vi "NM GlobalTest.vi"() -> ()   [LabVIEW 2010] (continued)
  in  "data 21":digitalwaveform[](array[waveform])
  in  "sDWrite":T7(tab)
  in  "data 22":bool
  in  "data 23":bool[](array[boolean])
  in  "data 24":u8 format="%x"
  in  "data 25":u16 format="%x"
  in  "data 26":u32 format="%x"
  in  "data 27":digitalwaveform(waveform)={"t0"=timestamp(0 s since 1904-01-01), "dt"=0.0, "Y"={"transitions"=[], "data"=[]}, "error"={"status"=FALSE, "code"=37421928, "source"=""}}
  out "data 28":u8[](array[numeric])
  out "data 29":u16[](array[numeric]) format="%x"
  out "data 30":u32[](array[numeric]) format="%x"
  in  "data 31":digitalwaveform(waveform)={"t0"=timestamp(0 s since 1904-01-01), "dt"=0.0, "Y"={"transitions"=[], "data"=[]}, "error"={"status"=FALSE, "code"=37421928, "source"=""}}
  in  "nOrsCChan":enum32{"Multi-Channel", "Single Channel"}(tab)=enum."Single Channel"
  in  "nCtrWrite":enum32{"Frequency", "Time", "Ticks"}(tab)
  in  "data 32":cluster{"duty cycle":dbl, "frequency":dbl}[](array[cluster])
  in  "data 34":cluster{"high time":dbl, "low time":dbl}[](array[cluster])
  in  "data 33":cluster{"high ticks":u32, "low ticks":u32}[](array[cluster])
  in  "sCtrWrite":enum32{"Frequency", "Time", "Ticks"}(tab)
  in  "frequency":dbl=1.0 format="%_6g"
  in  "duty cycle":dbl=0.5 format="%_6g"
  in  "high time":dbl=0.01 format="%_6g"
  in  "low time":dbl=0.01 format="%_6g"
  in  "high ticks":u32=100
  in  "low ticks":u32=100
  in  "CompWrite":enum32{"2D", "1D Waveform"}(tab)
  out "DblArray 2":dbl[][](array[numeric])
  out "u32Array":u32[][](array[numeric])
  out "DblPlot":dbl[][](graph)
  out "u32Plot":u32[][](graph)
  in  "Plots":bool
  in  "digital data 2":digitalwaveform[](array[waveform])
  out "WfmArray":waveform(dbl)[](array[waveform])
  in  "Write":bool
  in  "SelLib":enum32{"ULx", "DAQmx"}(tab)
  out "NumberOfChannels":u32
  out "Task":i32 format="%x"
  out "ToString":string
  out "ChanType":i32(ring)=10100 items=["Analog Input"=10100, "Analog Output"=10102, "Digital Input"=10151, "Digital Output"=10153, "Counter Input"=10131, "Counter Output"=10132]
  out "Name":refnum<k21>
  in  "Task Control Action":i32(ring)=2 items=["verify"=2, "reserve"=4, "commit"=3, "unreserve"=5, "abort"=6]
  in  "TaskType":T10(tab)
  in  "AChan":enum32{"ULx", "DAQmx"}(tab)
  in  "AnalogType":T11(tab)
  in  "min 3":dbl=-5.0
  in  "max 3":dbl=5.0
  in  "min 2":dbl=-5.0
  in  "max 2":dbl=5.0
  in  "min":dbl=-5.0
  in  "max":dbl=5.0
  in  "physical channels 3":refnum<k21>
  in  "physical channels 2":refnum<k21>
  in  "ULx":refnum<k21>
  in  "min 5":dbl=-0.01 format="%_4f"
  in  "max 5":dbl=0.01 format="%_4g"
  in  "min 4":dbl=-0.01 format="%_4f"
  in  "max 4":dbl=0.01 format="%_4g"
  in  "min":dbl=-0.01 format="%_4f"
  in  "max":dbl=0.01 format="%_4g"
  in  "physical channels 6":refnum<k21>
  in  "physical channels 5":refnum<k21>
  in  "ULx":refnum<k21>
  in  "units 3":i32(ring) items=["degC", "degF", "kelvin", "raw"]
  in  "units 2":i32(ring) items=["degC", "degF", "kelvin", "raw"]
  in  "units":i32(ring) items=["degC", "degF", "kelvin", "raw"]
  in  "physical channels 9":refnum<k21>
  in  "physical channels 8":refnum<k21>
  in  "ULx":refnum<k21>
  in  "physical channels 12":refnum<k21>
  in  "min 7":dbl=-5.0
  in  "max 7":dbl=5.0
  in  "physical channels 11":refnum<k21>
  in  "min 8":dbl=-5.0
  in  "max 8":dbl=5.0
  in  "min":dbl=-5.0
  in  "max":dbl=5.0
  in  "ULx":refnum<k21>
  in  "min 10":dbl=-10.0
  in  "max 10":dbl=10.0
  in  "min 11":dbl=-10.0
  in  "max 11":dbl=10.0
  in  "min":dbl=-10.0
  in  "max":dbl=10.0
  in  "physical channels 15":refnum<k21>
  in  "physical channels 14":refnum<k21>
  in  "ULx":refnum<k21>
  in  "xAnalog\nType":T11(tab)
  in  "physical channels 33":tag
  in  "physical channels 32":tag
  in  "DAQmx":tag
  in  "min 20":dbl=-5.0
  in  "max 20":dbl=5.0
  in  "min 19":dbl=-5.0
  in  "max 19":dbl=5.0
  in  "min":dbl=-5.0
  in  "max":dbl=5.0
  in  "name 1":string
  in  "name 2":string
  in  "name 3":string
  in  "physical channels 36":tag
  in  "physical channels 35":tag
  in  "min 23":dbl=-0.01 format="%0.5f"
  in  "max 23":dbl=0.01 format="%0.5f"
  in  "min 22":dbl=-0.01 format="%0.5f"
  in  "max 22":dbl=0.01 format="%0.5f"
  in  "min":dbl=-0.01 format="%0.5f"
  in  "max":dbl=0.01 format="%0.5f"
  in  "DAQmx":tag
  in  "units 15":i32(ring)=10143 items=["Deg C"=10143, "Deg F"=10144, "Kelvins"=10325, "Deg R"=10145, "From Custom Scale"=10065]
  in  "units 13":i32(ring)=10143 items=["Deg C"=10143, "Deg F"=10144, "Kelvins"=10325, "Deg R"=10145, "From Custom Scale"=10065]
  in  "min 26":dbl format="%0.2f"
  in  "max 26":dbl=100.0 format="%0.2f"
  in  "min 25":dbl format="%0.2f"
  in  "max 25":dbl=100.0 format="%0.2f"
  in  "min":dbl format="%0.2f"
  in  "max":dbl=100.0 format="%0.2f"
  in  "physical channels 39":tag
  in  "physical channels 38":tag
  in  "units":i32(ring)=10143 items=["Deg C"=10143, "Deg F"=10144, "Kelvins"=10325, "Deg R"=10145, "From Custom Scale"=10065]
  in  "DAQmx":tag
  in  "Names":string
  in  "T2":string
  in  "T3":string
  in  "min 29":dbl=-10.0 format="%0.2f"
  in  "max 29":dbl=10.0 format="%0.2f"
  in  "min 28":dbl=-10.0 format="%0.2f"
  in  "max 28":dbl=10.0 format="%0.2f"
  in  "min":dbl=-10.0 format="%0.2f"
  in  "max":dbl=10.0 format="%0.2f"
  in  "physical channels 42":tag
  in  "physical channels 41":tag
  in  "DAQmx":tag
  in  "physical channels 45":tag
  in  "physical channels 44":tag
  in  "min 32":dbl format="%0.5f"
  in  "max 32":dbl=0.02 format="%0.5f"
  in  "min 31":dbl format="%0.5f"
  in  "max 31":dbl=0.02 format="%0.5f"
  in  "min":dbl format="%0.5f"
  in  "max":dbl=0.02 format="%0.5f"
  in  "DAQmx":tag
  in  "DChan":enum32{"ULx", "DAQmx"}(tab)
  in  "DigitalType":enum32{"Digital Input", "Digital Output"}(tab)
  in  "line grouping 3":i32(ring)=1 items=["OneChannelForEachLine", "OneChannelForAllLines"]
  in  "line grouping 2":i32(ring)=1 items=["OneChannelForEachLine", "OneChannelForAllLines"]
  in  "line grouping":i32(ring)=1 items=["OneChannelForEachLine", "OneChannelForAllLines"]
  in  "lines 3":refnum<k21>
  in  "lines 2":refnum<k21>
  in  "ULx":refnum<k21>
  in  "line grouping 6":i32(ring)=1 items=["OneChannelForEachLine", "OneChannelForAllLines"]
  in  "line grouping 5":i32(ring)=1 items=["OneChannelForEachLine", "OneChannelForAllLines"]
  in  "line grouping":i32(ring)=1 items=["OneChannelForEachLine", "OneChannelForAllLines"]
  in  "lines 6":refnum<k21>
  in  "lines 5":refnum<k21>
  in  "ULx":refnum<k21>
  in  "xDigitalType":enum32{"Digital Input", "Digital Output"}(tab)
  in  "lines 9":tag
  in  "line grouping 8":i32(ring)=1 items=["one channel for each line", "one channel for all lines"]
  in  "line grouping 7":i32(ring)=1 items=["one channel for each line", "one channel for all lines"]
  in  "lines 8":tag
  in  "line grouping 4":i32(ring)=1 items=["one channel for each line", "one channel for all lines"]
  in  "DAQmx":tag
  in  "line grouping 11":i32(ring)=1 items=["one channel for each line", "one channel for all lines"]
  in  "lines 12":tag
  in  "line grouping 10":i32(ring)=1 items=["one channel for each line", "one channel for all lines"]
  in  "lines 11":tag
  in  "line grouping 9":i32(ring)=1 items=["one channel for each line", "one channel for all lines"]
  in  "DAQmx":tag
  in  "CtrChan":enum32{"ULx", "DAQmx"}(tab)
  in  "CounterType":T12(tab)
  in  "measure time 3":dbl=0.01 format="%.3f"
  in  "measure time 2":dbl=0.01 format="%.3f"
  in  "measure time":dbl=0.01 format="%.7f"
  in  "starting edge 3":i32(ring) items=["Rising", "Falling"]
  in  "starting edge 2":i32(ring) items=["Rising", "Falling"]
  in  "starting edge":i32(ring) items=["Rising", "Falling"]
  in  "units 6":i32(ring) items=["Hz", "Ticks"]
  in  "units 5":i32(ring) items=["Hz", "Ticks"]
  in  "units":i32(ring) items=["Hz", "Ticks"]
  in  "counters 3":refnum<k21>
  in  "counters 2":refnum<k21>
  in  "ULx":refnum<k21>
  in  "measure time 5":dbl=0.01 format="%.3f"
  in  "measure time 4":dbl=0.01 format="%.3f"
  in  "measure time":dbl=0.01 format="%.5f"
  in  "starting edge 6":i32(ring) items=["Rising", "Falling"]
  in  "starting edge 5":i32(ring) items=["Rising", "Falling"]
  in  "starting edge":i32(ring) items=["Rising", "Falling"]
  in  "units 9":i32(ring) items=["Seconds", "Ticks"]
  in  "units 8":i32(ring) items=["Seconds", "Ticks"]
  in  "units":i32(ring) items=["Seconds", "Ticks"]
  in  "counters 6":refnum<k21>
  in  "counters 5":refnum<k21>
  in  "ULx":refnum<k21>
  in  "edge 3":i32(ring) items=["Rising", "Falling"]
  in  "edge 2":i32(ring) items=["Rising", "Falling"]
  in  "edge":i32(ring) items=["Rising", "Falling"]
  in  "direction 3":i32(ring) items=["CountUp", "CountDown"]
  in  "direction 2":i32(ring) items=["CountUp", "CountDown"]
  in  "initial count 3":u32
  in  "direction":i32(ring) items=["CountUp", "CountDown"]
  in  "initial count 2":u32
  in  "initial count":u32
  in  "counters 9":refnum<k21>
  in  "counters 8":refnum<k21>
  in  "ULx":refnum<k21>
  in  "pulses per 2":u32=24
  in  "initial angle\npulses per":dbl
  in  "type 2":i32(ring)=2 items=["X1", "X2", "X4"]
  in  "index mode 2":i32(ring) items=["Disabled"=0, "LatchCounter"=8, "ResetCounter"=32]
  in  "units 11":i32(ring) items=["Degrees", "Radians", "Ticks"]
  in  "counters 11":refnum<k21>
  in  "initial angle\npulses per":dbl
  in  "pulses per":u32=24
  in  "type":i32(ring)=2 items=["X1", "X2", "X4"]
  in  "index mode":i32(ring) items=["Disabled"=0, "LatchCounter"=8, "ResetCounter"=32]
  in  "units 10":i32(ring) items=["Degrees", "Radians", "Ticks"]
  in  "ULx":refnum<k21>
  in  "duty cycle 3":dbl=0.5 format="%.6f"
  in  "duty cycle 2":dbl=0.5 format="%.6f"
  in  "frequency 3":dbl=1.0 format="%.6f"
  in  "frequency 2":dbl=1.0 format="%.6f"
  in  "duty cycle":dbl=0.5 format="%.6f"
  in  "frequency":dbl=1.0 format="%.6f"
  in  "counters 14":refnum<k21>
  in  "counters 13":refnum<k21>
  in  "ULx":refnum<k21>
  in  "low time 3":dbl=0.01 format="%.6f"
  in  "high time 3":dbl=0.01 format="%.6f"
  in  "low time 2":dbl=0.01 format="%.6f"
  in  "high time 2":dbl=0.01 format="%.6f"
  in  "low time":dbl=0.01 format="%.8f"
  in  "high time":dbl=0.01 format="%.8f"
  in  "counters 19":refnum<k21>
  in  "counters 18":refnum<k21>
  in  "ULx":refnum<k21>
  in  "low ticks 3":u32=100
  in  "high ticks 3":u32=100
  in  "low ticks 2":u32=100
  in  "high ticks 2":u32=100
  in  "low ticks":u32=100
  in  "high ticks":u32=100
  in  "counters 20":refnum<k21>
  in  "counters 16":refnum<k21>
  in  "ULx":refnum<k21>
  in  "xCntrType":T12(tab)
  in  "FreqChan":enum32{"Chan 1", "Chan 2", "Chan 3"}(tab)
  in  "divisor":u32=4
  in  "measurement method":i32(ring)=10105 items=["Low Frequency with 1 Counter"=10105, "High Frequency with 2 Counters"=10157, "Large Range with 2 Counters"=10205]
  in  "start edge":i32(ring)=10280 items=["Rising"=10280, "Falling"=10171]
  in  "units":i32(ring)=10373 items=["Hz"=10373, "Ticks"=10304, "From Custom Scale"=10065]
  in  "min":dbl=2.0 format="%0.6f"
  in  "max":dbl=100.0 format="%0.6f"
  in  "DAQmx":tag
  in  "measurement time":dbl=0.001 format="%0.6f"
  in  "DAQmx":tag
  in  "max":dbl=100.0 format="%0.6f"
  in  "min 21":dbl=2.0 format="%0.6f"
  in  "measurement method":i32(ring)=10105 items=["Low Frequency with 1 Counter"=10105, "High Frequency with 2 Counters"=10157, "Large Range with 2 Counters"=10205]
  in  "start edge":i32(ring)=10280 items=["Rising"=10280, "Falling"=10171]
  in  "divisor 5":u32=4
  in  "units":i32(ring)=10373 items=["Hz"=10373, "Ticks"=10304, "From Custom Scale"=10065]
  in  "measurement time 2":dbl=0.001 format="%0.6f"
  in  "DAQmx":tag
  in  "max":dbl=100.0 format="%0.6f"
  in  "min 24":dbl=2.0 format="%0.6f"
  in  "start edge":i32(ring)=10280 items=["Rising"=10280, "Falling"=10171]
  in  "measurement method":i32(ring)=10105 items=["Low Frequency with 1 Counter"=10105, "High Frequency with 2 Counters"=10157, "Large Range with 2 Counters"=10205]
  in  "units":i32(ring)=10373 items=["Hz"=10373, "Ticks"=10304, "From Custom Scale"=10065]
  in  "divisor 6":u32=4
  in  "measurement time 3":dbl=0.001 format="%0.6f"
  in  "PerChan":enum32{"Chan 1", "Chan 2", "Chan 3"}(tab)
  in  "DAQmx":tag
  in  "measure time 6":dbl=0.001 format="%0.6f"
  in  "measurement method":i32(ring)=10105 items=["Low Frequency with 1 Counter"=10105, "High Frequency with 2 Counters"=10157, "Large Range with 2 Counters"=10205]
  in  "max":dbl=0.1 format="%0.6f"
  in  "min":dbl=1e-06 format="%0.6f"
  in  "start edge":i32(ring)=10280 items=["Rising"=10280, "Falling"=10171]
  in  "divisor":u32=4
  in  "units":i32(ring)=10364 items=["Seconds"=10364, "Ticks"=10304, "From Custom Scale"=10065]
  in  "DAQmx":tag
  in  "max":dbl=0.1 format="%0.6f"
  in  "min":dbl=1e-06 format="%0.6f"
  in  "start edge":i32(ring)=10280 items=["Rising"=10280, "Falling"=10171]
  in  "measurement method":i32(ring)=10105 items=["Low Frequency with 1 Counter"=10105, "High Frequency with 2 Counters"=10157, "Large Range with 2 Counters"=10205]
  in  "units":i32(ring)=10364 items=["Seconds"=10364, "Ticks"=10304, "From Custom Scale"=10065]
  in  "measure time 7":dbl=0.001 format="%0.6f"
  in  "divisor 2":u32=4
  in  "DAQmx":tag
  in  "max":dbl=0.1 format="%0.6f"
  in  "min":dbl=1e-06 format="%0.6f"
  in  "start edge":i32(ring)=10280 items=["Rising"=10280, "Falling"=10171]
  in  "measurement method":i32(ring)=10105 items=["Low Frequency with 1 Counter"=10105, "High Frequency with 2 Counters"=10157, "Large Range with 2 Counters"=10205]
  in  "units":i32(ring)=10364 items=["Seconds"=10364, "Ticks"=10304, "From Custom Scale"=10065]
  in  "measure time 8":dbl=0.001 format="%0.6f"
  in  "divisor 3":u32=4
  in  "edge 8":i32(ring)=10280 items=["Rising"=10280, "Falling"=10171]
  in  "direction 8":i32(ring)=10128 items=["Count Up"=10128, "Count Down"=10124, "Externally Controlled"=10326]
  in  "init count 3":u32
  in  "edge 7":i32(ring)=10280 items=["Rising"=10280, "Falling"=10171]
  in  "direction 7":i32(ring)=10128 items=["Count Up"=10128, "Count Down"=10124, "Externally Controlled"=10326]
  in  "init count 2":u32
  in  "counter 9":tag
  in  "counter 8":tag
  in  "edge":i32(ring)=10280 items=["Rising"=10280, "Falling"=10171]
  in  "direction":i32(ring)=10128 items=["Count Up"=10128, "Count Down"=10124, "Externally Controlled"=10326]
  in  "init count":u32
  in  "DAQmx":tag
  in  "type":i32(ring)=10092 items=["X1"=10090, "X2"=10091, "X4"=10092, "Two Pulse Counting"=10313]
  in  "type":i32(ring)=10092 items=["X1"=10090, "X2"=10091, "X4"=10092, "Two Pulse Counting"=10313]
  in  "pulses per revolution 2":u32=24
  in  "initial angle\npulses per":dbl
  in  "units 22":i32(ring)=10146 items=["Degrees"=10146, "Radians"=10273, "Ticks"=10304, "From Custom Scale"=10065]
  in  "z phase 2":i32(ring)=10040 items=["A High B High"=10040, "A High B Low"=10041, "A Low B High"=10042, "A Low B Low"=10043]
  in  "z value 2":dbl
  in  "z index  2":bool
  in  "counter 11":tag
  in  "pulses per revolution":u32=24
  in  "initial angle\npulses per":dbl
  in  "z phase":i32(ring)=10040 items=["A High B High"=10040, "A High B Low"=10041, "A Low B High"=10042, "A Low B Low"=10043]
  in  "z value":dbl
  in  "z index":bool
  in  "units":i32(ring)=10146 items=["Degrees"=10146, "Radians"=10273, "Ticks"=10304, "From Custom Scale"=10065]
  in  "DAQmx":tag
  in  "initial delay 4":dbl format="%.6f"
  in  "idle state 4":i32(ring)=10214 items=["High"=10192, "Low"=10214]
  in  "initial delay 5":dbl format="%.6f"
  in  "idle state 5":i32(ring)=10214 items=["High"=10192, "Low"=10214]
  in  "duty cycle 6":dbl=0.5 format="%.6f"
  in  "frequency 6":dbl=1.0 format="%.6f"
  in  "counter 14":tag
  in  "counter 13":tag
  in  "duty cycle 5":dbl=0.5 format="%.6f"
  in  "frequency 5":dbl=1.0 format="%.6f"
  in  "initial delay":dbl format="%.6f"
  in  "idle state":i32(ring)=10214 items=["High"=10192, "Low"=10214]
  in  "duty cycle":dbl=0.5 format="%.6f"
  in  "frequency":dbl=1.0 format="%.6f"
  in  "DAQmx":tag
  in  "low time 6":dbl=0.01 format="%.6f"
  in  "high time 6":dbl=0.01 format="%.6f"
  in  "low time 5":dbl=0.01 format="%.6f"
  in  "high time 5":dbl=0.01 format="%.6f"
  in  "idle state":i32(ring)=10214 items=["High"=10192, "Low"=10214]
  in  "low time":dbl=0.01 format="%.6f"
  in  "high time":dbl=0.01 format="%.6f"
  in  "initial delay 7":dbl format="%.6f"
  in  "idle state 8":i32(ring)=10214 items=["High"=10192, "Low"=10214]
  in  "initial delay 8":dbl format="%.6f"
  in  "idle state 9":i32(ring)=10214 items=["High"=10192, "Low"=10214]
  in  "counter 17":tag
  in  "counter 16":tag
  in  "initial delay":dbl format="%.6f"
  in  "DAQmx":tag
  in  "TickChan":enum32{"Chan 1", "Chan 2", "Chan 3"}(tab)
  in  "source of ticks":tag="OnboardClock"
  in  "DAQmx":tag
  in  "low ticks":u32=100
  in  "high ticks":u32=100
  in  "idle state":i32(ring)=10214 items=["High"=10192, "Low"=10214]
  in  "initial delay":u32
  in  "idle state":i32(ring)=10214 items=["High"=10192, "Low"=10214]
  in  "DAQmx":tag
  in  "high ticks":u32=100
  in  "low ticks":u32=100
  in  "source of ticks":tag="OnboardClock"
  in  "initial delay":u32
  in  "idle state":i32(ring)=10214 items=["High"=10192, "Low"=10214]
  in  "DAQmx":tag
  in  "high ticks":u32=100
  in  "low ticks":u32=100
  in  "source of ticks":tag="OnboardClock"
  in  "initial delay":u32
  in  "CompIn":enum32{"ULx", "DAQmx"}(tab)
  in  "CompType":T13(tab)
  in  "min 12":dbl=-5.0
  in  "max 12":dbl=5.0
  in  "min 9":dbl=-5.0
  in  "max 9":dbl=5.0
  in  "min":dbl=-5.0
  in  "max":dbl=5.0
  in  "physical channels 18":refnum<k21>
  in  "physical channels 17":refnum<k21>
  in  "ULx":refnum<k21>
  in  "units 12":i32(ring) items=["degC", "degF", "kelvin", "raw"]
  in  "units 7":i32(ring) items=["degC", "degF", "kelvin", "raw"]
  in  "units":i32(ring) items=["degC", "degF", "kelvin", "raw"]
  in  "physical channels 21":refnum<k21>
  in  "physical channels 20":refnum<k21>
  in  "ULx":refnum<k21>
  in  "ports 3":refnum<k21>
  in  "ports 2":refnum<k21>
  in  "ULx":refnum<k21>
  in  "edge 6":i32(ring) items=["Rising", "Falling"]
  in  "direction 6":i32(ring) items=["CountUp", "CountDown"]
  in  "initial count 6":u32
  in  "edge 5":i32(ring) items=["Rising", "Falling"]
  in  "direction 5":i32(ring) items=["CountUp", "CountDown"]
  in  "initial count 5":u32
  in  "edge":i32(ring) items=["Rising", "Falling"]
  in  "direction":i32(ring) items=["CountUp", "CountDown"]
  in  "initial count":u32
  in  "counters 23":refnum<k21>
  in  "counters 22":refnum<k21>
  in  "ULx":refnum<k21>
  in  "initial angle\npulses per":dbl
  in  "pulses per 4":dbl=24.0
  in  "type 4":dbl(ring)=2.0 items=["X1", "X2", "X4"]
  in  "z index mode 2":i32(ring) items=["Disabled"=0, "LatchCounter"=8, "ResetCounter"=32]
  in  "units 14":i32(ring) items=["Degrees", "Radians", "Ticks"]
  in  "initial angle\npulses per":dbl
  in  "pulses per 3":dbl=24.0
  in  "type":dbl(ring)=2.0 items=["X1", "X2", "X4"]
  in  "z index mode":i32(ring) items=["Disabled"=0, "LatchCounter"=8, "ResetCounter"=32]
  in  "units":i32(ring) items=["Degrees", "Radians", "Ticks"]
  in  "counters 25":refnum<k21>
  in  "ULx":refnum<k21>
  in  "ULx":refnum<k21>
  in  "physical channels 29":refnum<k21>
  in  "physical channels 30":refnum<k21>
  in  "max":dbl=5.0
  in  "min":dbl=-5.0
  in  "max 15":dbl=5.0
  in  "min 15":dbl=-5.0
  in  "max 18":dbl=5.0
  in  "min 18":dbl=-5.0
  in  "CompOut":enum32{"ULx", "DAQmx"}(tab)
  in  "CompOType":enum32{"AO Volts", "Digital Out", "AO Volts 2"}(tab)
  in  "min 14":dbl=-5.0
  in  "max 14":dbl=5.0
  in  "min 13":dbl=-5.0
  in  "max 13":dbl=5.0
  in  "min":dbl=-5.0
  in  "max":dbl=5.0
  in  "physical channels 24":refnum<k21>
  in  "physical channels 23":refnum<k21>
  in  "ULx":refnum<k21>
  in  "ports 6":refnum<k21>
  in  "ports 5":refnum<k21>
  in  "ULx":refnum<k21>
  in  "min 17":dbl=-5.0
  in  "max 17":dbl=5.0
  in  "min 16":dbl=-5.0
  in  "max 16":dbl=5.0
  in  "min":dbl=-5.0
  in  "max":dbl=5.0
  in  "physical channels 27":refnum<k21>
  in  "physical channels 26":refnum<k21>
  in  "ULx":refnum<k21>
  out "# of Loops":i32
  in  "Status\nLoop":bool
  out "Task Cleared":bool
  out "Task Stopped":bool
  in  "TrigType":enum32{"Basic", "Gated", "Start", "Stop"}(tab)
  in  "BasicType":T14(tab)
  in  "TrgEdge":enum32{"ULx", "DAQmx"}(tab)
  in  "ULx edge":i32(ring) items=["Rising", "Falling"]
  in  "pretrigger samples per channel":u32
  in  "DAQmx edge":i32(ring)=10280 items=["Rising"=10280, "Falling"=10171]
  in  "DAQmx source":tag
  in  "pretrigger samples per channel":u32
  in  "level":i32(ring)=1 items=["Low", "High"]
  in  "trig chan":refnum<k21>
  in  "sensitivity":i32(ring)=2 items=["AbovePattern", "BelowPattern", "EqualPattern", "NotEqualPattern"]
  in  "pattern":u64=32768 format="%04x"
  in  "mask":u64=65535 format="%04x"
  in  "Pretrig Samps":u32
  in  "pretrigger samples per channel":u32
  in  "level":dbl
  in  "slope":i32(ring) items=["Rising", "Falling"]
  in  "GatedType":T15(tab)
  in  "Level 3":i32(ring) items=["High", "Low"]
  in  "level":dbl
  in  "position":i32(ring) items=["Above", "Below"]
  in  "top":dbl=0.5
  in  "bottom":dbl
  in  "When":i32(ring) items=["InsideWindow", "OutsideWindow"]
  in  "hyst":i32(ring) items=["Negative", "Positive"]
  in  "low":dbl
  in  "high":dbl=0.5
  in  "StartType":T16(tab)
  in  "trigger sensitivity":i32(ring) items=["RisingEdge", "FallingEdge"]
  in  "variance":dbl
  in  "Level":dbl
  in  "sensitivity":i32(ring) items=["AboveLevel", "BelowLevel", "RisingEdge", "FallingEdge"]
  in  "trigger channel":refnum<k21>
  in  "pretrigger samples":u32
  in  "variance":dbl
  in  "Level":dbl
  in  "sensitivity":i32(ring) items=["AboveLevel", "BelowLevel", "RisingEdge", "FallingEdge"]
  in  "trigger channel":refnum<k21>
  in  "pretrigger samples":u32
  in  "variance":dbl
  in  "level":dbl
  in  "trigger sensitivity":i32(ring) items=["AboveLevel", "BelowLevel", "EqualLevel", "NotEqualLevel"]
  in  "trigger channel":refnum<k21>
  in  "pretrigger samples":u32
  in  "variance":dbl
  in  "level":dbl
  in  "trigger sensitivity":i32(ring) items=["AboveLevel", "BelowLevel", "EqualLevel", "NotEqualLevel"]
  in  "StopType":enum32{"None", "ASftwr", "DPtrn", "Ctr"}(tab)
  in  "trigger channel":refnum<k21>
  in  "variance":dbl
  in  "level":dbl
  in  "trigger sensitivity":i32(ring) items=["AboveLevel", "BelowLevel", "EqualLevel", "NotEqualLevel", "RisingEdge", "FallingEdge"]
  in  "trigger channel":refnum<k21>
  in  "level":dbl
  in  "variance":dbl
  in  "trigger sensitivity":i32(ring) items=["AboveLevel", "BelowLevel", "EqualLevel", "NotEqualLevel", "RisingEdge", "FallingEdge"]
  in  "trigger channel":refnum<k21>
  in  "trigger sensitivity":i32(ring) items=["AboveLevel", "BelowLevel", "EqualLevel", "NotEqualLevel", "RisingEdge", "FallingEdge"]
  in  "level":dbl
  in  "variance":dbl
  in  "Trig":bool caption="(F5)"
  in  "Start":bool
  in  "Timing":bool caption="(F4)"
  in  "Tab Control":enum32{"Clock", "Waveform", "Implicit"}(tab)
  in  "UDClock":enum32{"ULx", "DAQmx"}(tab)
  in  "samples per":i32=1000 format="%#.4p"
  in  "sample mode":i32(ring) items=["FiniteSamples", "ContinuousSamples"]
  in  "clock source":i32(ring) items=["OnboardClock", "ExternalClock", "NoClock"]
  in  "rate":dbl=1000.0 format="%#.4p"
  in  "mxRate":dbl=1000.0 format="%0.2f"
  in  "sample mode":i32(ring)=10178 items=["Finite Samples"=10178, "Continuous Samples"=10123, "Hardware Timed Single Point"=12522]
  in  "samples per":i32=1000
  in  "source":tag="OnboardClock"
  in  "active edge":i32(ring)=10280 items=["Rising"=10280, "Falling"=10171]
  in  "TmgWfm":enum32{"ULx", "DAQmx"}(tab)
  in  "waveform":waveform(dbl)={"t0"=timestamp(0 s since 1904-01-01), "dt"=0.0, "Y"=[]}
  in  "sample mode 3":i32(ring) items=["FiniteSamples", "ContinuousSamples"]
  in  "waveform 2":waveform(dbl)={"t0"=timestamp(0 s since 1904-01-01), "dt"=0.0, "Y"=[]}
  in  "sample mode 2":i32(ring)=10178 items=["Finite Samples"=10178, "Continuous Samples"=10123, "Hardware Timed Single Point"=12522]
  in  "TmgImp":enum32{"ULx", "DAQmx"}(tab)
  in  "samples per channel":i32=1000
  in  "sample mode":i32(ring) items=["FiniteSamples", "ContinuousSamples"]
  in  "sample mode":i32(ring)=10178 items=["Finite Samples"=10178, "Continuous Samples"=10123, "Hardware Timed Single Point"=12522]
  in  "samples per channel":i32=1000
  out "Idle":bool
  in  "Idle":bool=TRUE
  in  "Submit":bool
  in  "stop":bool
  in  "Stop":bool
  in  "Clear":bool
  out "message 2":string
  # "Current Task"
  # "Delays"
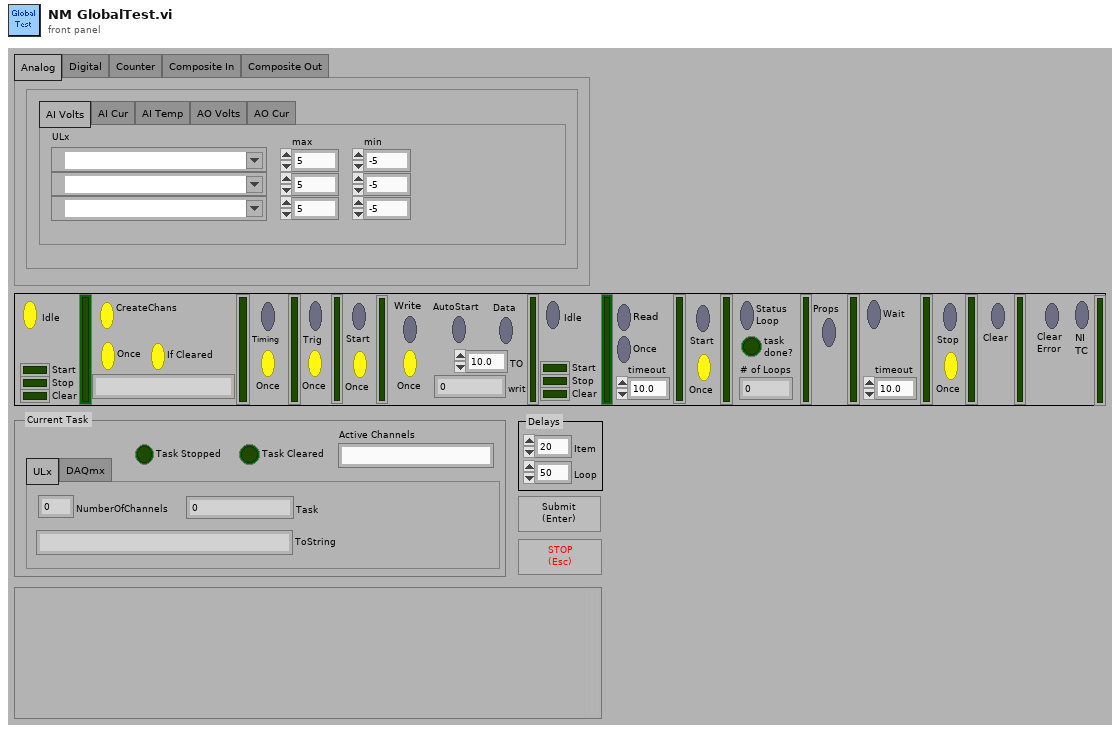
[diagram p1: front panel]
types:
  T1 = enum16{"Sine Wave", "Triangle Wave", "Square Wave", "Sawtooth Wave"}
  T2 = enum32{"Read", "Write", "Trigger", "Timing", "AI", "CI", "CO"}
  T3 = enum32{"Frequency", "Period", "Edges", "Encoder"}
  T4 = enum32{"Analog", "Digital", "Counter", "Composite"}
  T5 = enum32{"sCsSDbl", "sCsSWfm", "sCnS1D", "sCnSWfm", "nCsSDbl", "nCsSWfm", "nCnS2D", "nCnS1DWfm", "2DI16", "2DI32", "2DU16", "2DU32"}
  T6 = enum32{"nCsSBool", "nCsS2D", "nCsSU8", "nCsSU16", "nCsSU32", "nCsSWv", "nCnSU8", "nCnSU16", "nCnSU32", "nCnSWv"}
  T7 = enum32{"sCsSBool", "sCsS1D", "sCsSU8", "sCsSU16", "sCsSU32", "sCsSWv", "sCnSU8", "sCnSU16", "sCnSU32", "sCnSWv"}
  T8 = enum32{"sCsSDbl", "sCsSU32", "sCnSDbl", "sCnSU32", "nCsSDbl", "nCsSU32", "nCnSDbl", "nCnSU32"}
  T9 = enum32{"sCsSDbl", "sCsSWfm", "sCnS1D", "sCnSWfm", "nCsSDbl", "nCsSWfm", "nCnS2D", "nCnS1DWfm", "2DI16", "2DI32", "2DU16"}
  T10 = enum32{"Analog", "Digital", "Counter", "Composite In", "Composite Out"}
  T11 = enum32{"AI Volts", "AI Cur", "AI Temp", "AO Volts", "AO Cur"}
  T12 = enum32{"Freq In", "Period In", "Edge In", "Position In", "Freq Out", "Time Out", "Ticks Out"}
  T13 = enum32{"AI Volts", "AI Temp", "Digital In", "Counter In", "Encoder In", "AI Volts 2"}
  T14 = enum32{"None", "DEdge", "DLevel", "DPtrn", "AEdge"}
  T15 = enum32{"None", "DLevel", "ALevel", "AWindow", "AHyst"}
  T16 = enum32{"None", "ExtTTL", "AHdwr", "ASftwr", "DPtrn", "Ctr"}
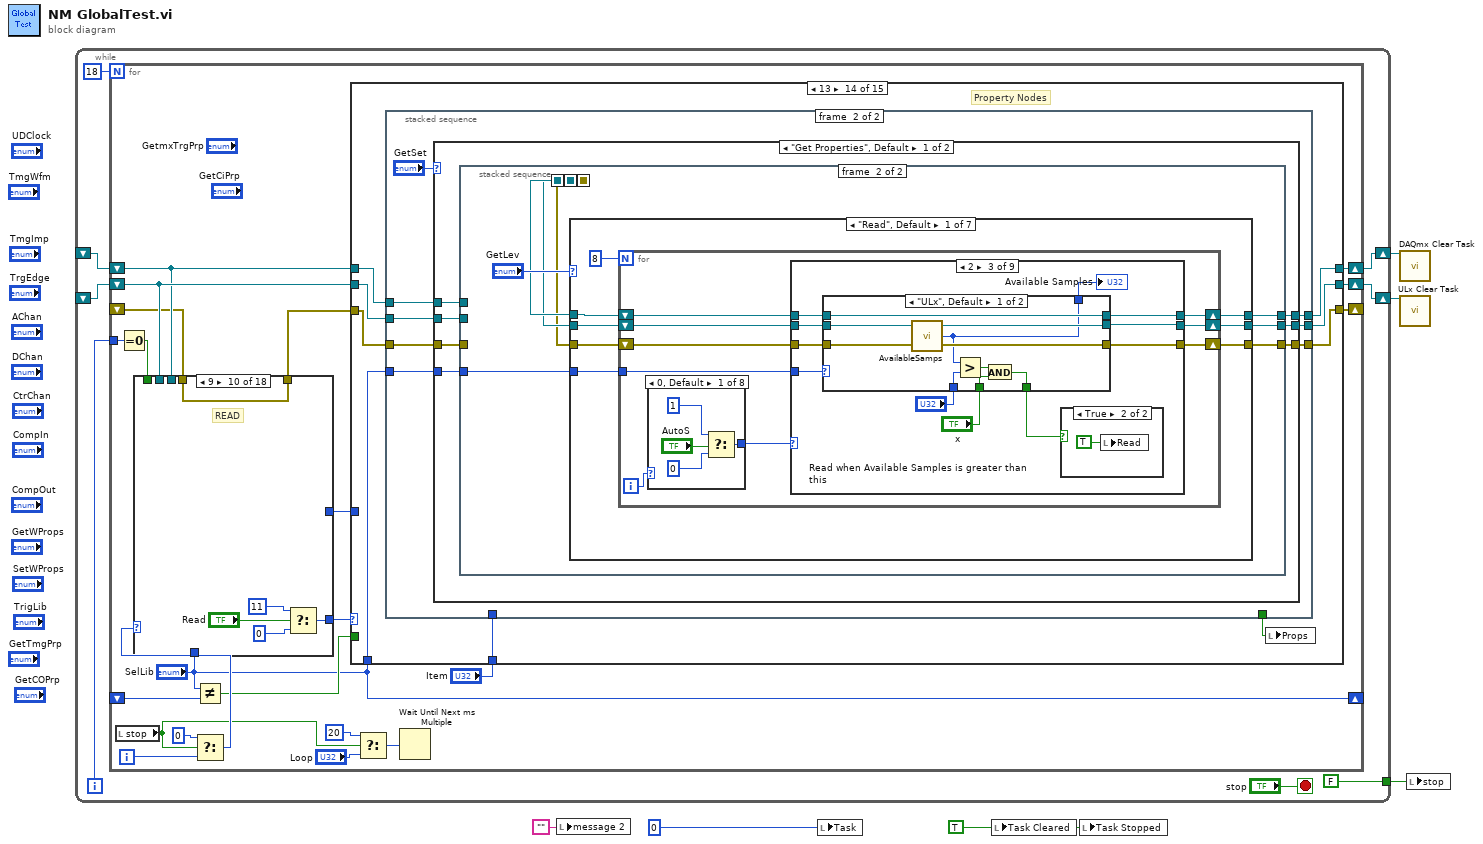
[diagram p0: block diagram]
diagram:
  w5 = TRUE ("Task Cleared")
  n1 = while {
    tunnel: [FALSE ("stop")] -> w6
    shift-right: [w11] -> w3
    shift-left: _ -> [w8]
    shift-right: [w10] -> w2
    shift-left: _ -> [w7]
    i -> [w12]
    stop <- "stop" stop-if-true
    n2 = for {
      N: 18 -> [_]
      tunnel: w12 -> [w36]
      shift-right: [w32] -> _
      shift-left: _ -> [w21]
      shift-right: [w35] -> w11
      shift-left: w8 -> [w22]
      shift-right: [w34] -> w10
      shift-left: w7 -> [w23]
      shift-right: ["SelLib"] -> _
      shift-left: _ -> [w18]
      i -> [w30]
      n3 = local read "stop"() -> (w25:bool)
      n4 = Equal To 0?(x=w36) -> (x = 0?=w24:bool)
      n5 = Not Equal?(x="SelLib", y=w18) -> (x != y?=w17:bool)
      n6 = Select(t=0, s=w25, f=w30) -> (s? t:f=w29:i32)
      n7 = case shown="9" w29 {
        tunnel: [0 ("f") w5815 w5830 3 ("f") w5836 w5841 w5846 w5851 w5856 w5861 w5867 w5873 w5877 w5882 w5888 w5897 w5904 0 ("f")] -> w33
        tunnel: w24 -> [_ _ w5823 _ _ _ _ _ _ _ _ _ _ _ _ _ _ _]
        tunnel: w23 -> [w5805 _ _ _ _ _ _ _ _ _ _ _ _ _ _ w5894 _ _]
        tunnel: "SelLib" -> [w5804 _ _ _ _ _ _ _ _ _ _ _ _ _ _ w5893 _ _]
        tunnel: w22 -> [w5803 _ _ _ _ _ _ _ _ _ _ _ _ _ _ w5895 _ _]
        tunnel: w21 -> [w5801 w5812 w5818 w5833 w5834 w5839 w5844 w5849 w5854 w5860 w5865 w5871 w5876 w5881 w5886 w5891 w5908 w5910]
        tunnel: [_ 0 ("f") _ _ _ _ _ _ 1 ("f") _ 1 ("f") _ _ _ _ _ _ _] -> w19
        tunnel: [w5801 w5812 w5818 w5833 w5834 w5839 w5844 w5849 w5854 w5860 w5865 w5871 w5876 w5881 w5886 w5891 w5908 w5909] -> w16
        frame 0, Default {
          # "Do Nothing"
          n8 = case shown="\"ULx\", Default" w5804 {
            tunnel: w5805 -> [w5809 _]
            tunnel: w5803 -> [_ w5811]
            tunnel: [w5807 w5810] -> w5802
            frame "ULx", Default {
              n9 = call "ULxTaskInfo.vi"("task in"=w5809) -> ("Task"=w5808:i32)  [unwired: 2 out]
              n10 = Equal To 0?(x=w5808) -> (x = 0?=w5807:bool)
            }
            frame "DAQmx" {
              n11 = call "mxTaskCleared.vi"("task in"=w5811) -> ("Task Cleared"=w5810:bool)
            }
          }
          n12 = local write "Task Cleared"(w5802) -> ()
        }
        frame 1 {
          # "IDLE and UPDATE CONTROLS"
          n13 = Select(t=1, s="Idle", f=0) -> (s? t:f=w5815:i32)
        }
        frame 2 {
          # "CREATE CHANNELS"
          n14 = local read "Task Cleared"() -> (w5828:bool)
          n15 = And(x=w5828, y="If Cleared") -> (x .and. y?=w5824:bool)
          n16 = Not(x="Once") -> (.not. x?=w5825:bool)
          n17 = Compound Arithmetic op=OR(w5823, w5824, w5825) -> (w5820:bool)
          n18 = Select(t=2, s=w5820, f=0) -> (s? t:f=w5819:i32)
          n19 = Select(t=w5819, s="CreateChans", f=0) -> (s? t:f=w5830:i32)
        }
        frame 3 {
          # "Channel Info"
        }
        frame 4 {
          # "TIMING"
